vi "OdorSystem-V2.vi"() -> ()   [LabVIEW 2019]
doc: "Synchronize Correlated Digital Output with Analog Input Using NI-DAQmx \n\nOverview:\nThis example uses DAQmx to synchronize finite generation and acquisition of Correlated Digital Output with an Analog Input Task respectively.\n\nDescriptions:\nCorrelated I/O enables synchronization of on board digital I/O lines to a clock reference. Digital and Analog samples can be synchronized in time by sharing the AI clock as the source of your digital I/O clock. You may also use the Counter Output pulse as the Source of Digital Timing. Hence, set the Source for Digital Timing as ai/SampleClock.This example will work on any device that uses DAQmx and supports Correlated Digital I/O. To perform Correlated Digital I/O on 9172 Chassis, you need a Correlated Module in slot 1-4 of the chassis. \n\nRequirements:\n1. LabVIEW 2012 or compatible.\n2. NI-DAQmx 15.5.1 or compatible.\n\nInstructions:\n1. Set all the control values on the front panel corresponding to the physical channel to be used on the DAQ device.\n2. Run this VI.\n3. Monitor the analog input voltage measured and ramp signal generated from specified channels. \n\nBlock Diagram Steps:\n1. Creates channels to measure voltage and to generate digital signals \n2. Sets the source of the Sample Clock, the rate of the Sample Clock, and the number of samples to acquire or generate.\n3. Generates an array containing a ramp pattern and write to digital output lines.\n4. Transitions the tasks to running state to begin measuring and generating data.\n5. Reads the waveform from the analog input channel and waits for the digital output generation to complete.\n6. Clears the tasks.\n7. Displays any error occurs."
uses:
  StatesEnum.ctl
  <vilib>/DAQmx/write.llb/DAQmx Write (Digital 1D Bool NChan 1Samp 1Line).vi
  <vilib>/DAQmx/write.llb/DAQmx Write (Digital Wfm 1Chan NSamp).vi
  <vilib>/DAQmx/read.llb/DAQmx Read (Counter 1D U32 1Chan NSamp).vi
  <vilib>/DAQmx/read.llb/DAQmx Read (Digital 1D Bool 1Chan 1Samp).vi
  <vilib>/DAQmx/miscellaneous.llb/DAQmx Fill In Error Info.vi
  <vilib>/DAQmx/create/channels.llb/DAQmx Create Channel (CO-Pulse Generation-Frequency).vi
  <vilib>/DAQmx/configure/timing.llb/DAQmx Timing (Implicit).vi
  <vilib>/Waveform/DWDTOps.llb/Digital Pattern Generator (Single Value).vi
  <vilib>/Waveform/DWDTOps.llb/DWDT Append Digital Samples.vi
  <vilib>/DAQmx/create/channels.llb/DAQmx Create Channel (CI-Count Edges).vi
  <vilib>/DAQmx/configure/timing.llb/DAQmx Timing (Sample Clock).vi
  <vilib>/Waveform/DWDTOps.llb/DWDT Append Digital Signals.vi
  <vilib>/Waveform/DWDTOps.llb/DWDT Digital to Boolean Array.vi
  <vilib>/DAQmx/create/channels.llb/DAQmx Create Channel (DO-Digital Output).vi
  <vilib>/Waveform/DWDTOps.llb/DWDT Uncompress Digital.vi
  <resource>/objmgr/daqmx.rc
panel:
  in  "Use Default vavle":bool=TRUE
  in  "Selected default valve":u8(knob)=8 min=1 max=8 step=1 scale=1.0..8.0
  out "Framecount":u32
  in  "Image count filepath":path
  out "Experiment running":bool
  out "State":T1
  in  "Select experiment":enum32{"Single trial", "Trial series"}(tab)
  out "Time elapsed":dbl format="%.1f"
  in  "Start single trial":bool
  out "single trial done":bool
  in  "Select valve":u8(knob)=1 min=1 max=8 step=1 scale=1.0..8.0
  out "Pause elapsed time":dbl format="%#.1f"
  out "In between trials":bool
  out "Trial elapsed time":dbl format="%.1f"
  out "Total elapsed time":dbl format="%.1f"
  out "Estimated total time":dbl
  out "Current list index":i32
  out "Current Valve":u8
  in  "Time between trials":u16=10 min=1 max=900 step=1
  in  "Start trial series":bool
  in  "Valve order list":i8[](array[numeric]) min=1 max=8 step=1
  out "Digitaler output":digitalwaveform(graph)
  out "Stop Boolesch":bool
  in  "Total trial time":dbl=20.0 min=1.0 step=0.1
  in  "Valve opening Time":dbl=10.0 min=0.0 step=0.1
  in  "Valve delay":dbl=2.0 min=0.0 step=0.1
  in  "Stopp":bool
  out "Digital Waveform Graph":digitalwaveform(graph)
  # "All times are in second!"
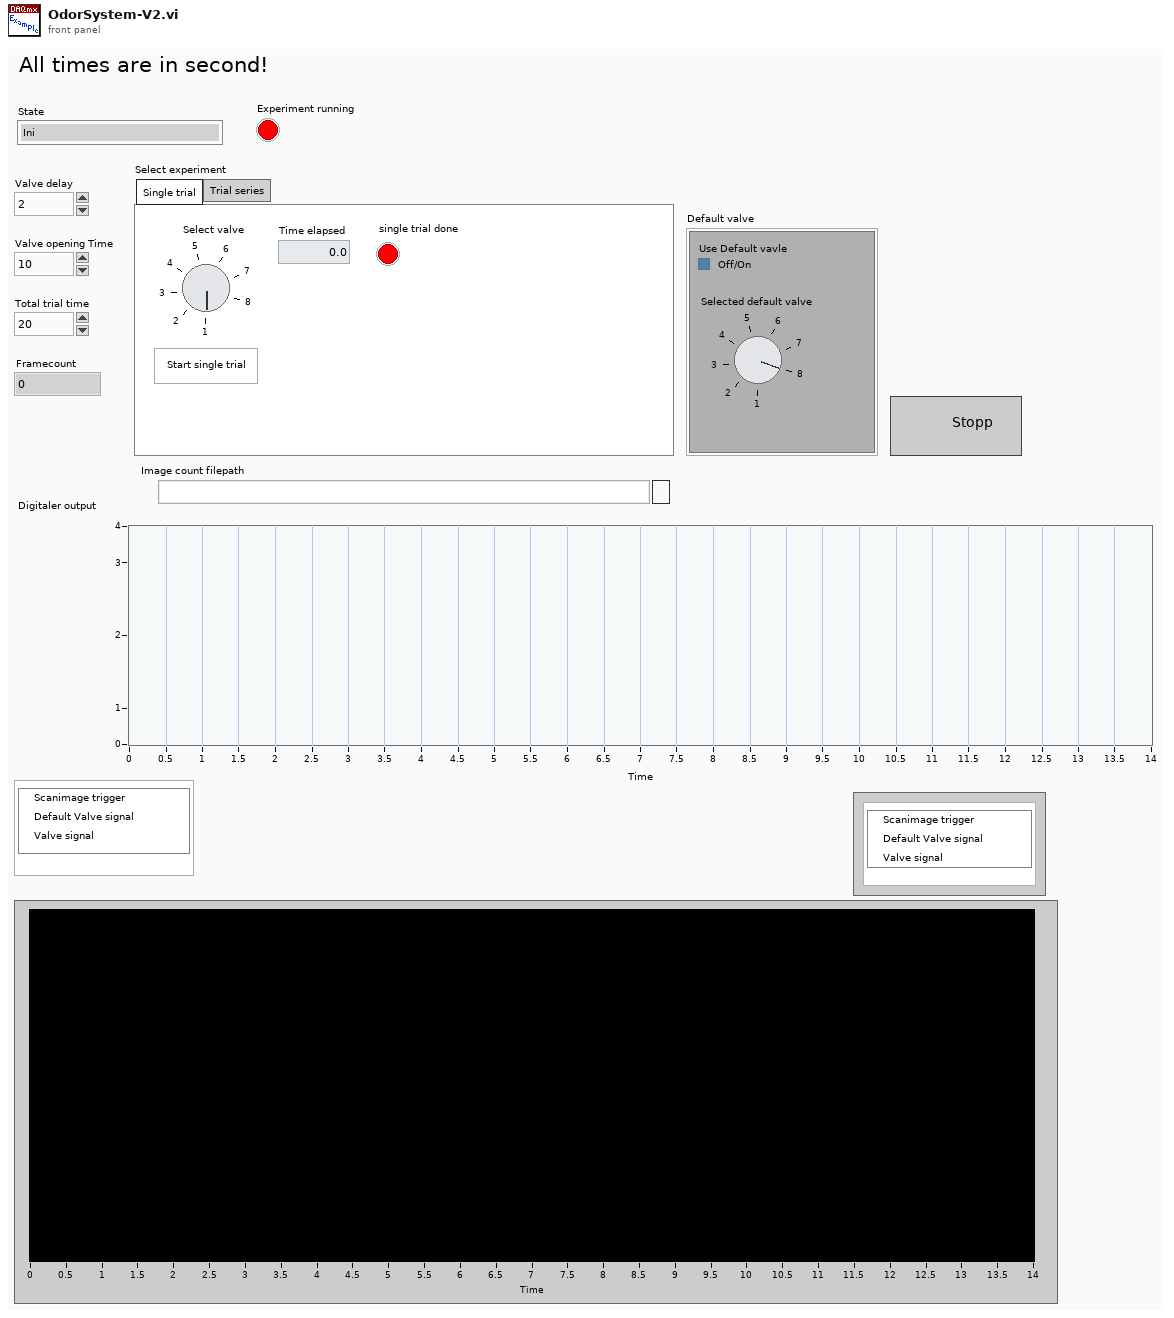
[diagram p1: front panel]
types:
  T1 = typedef "StatesEnum.ctl" = enum16{"Ini", "Standby", "Start Trial", "Start trial series", "Stop"}
  T2 = enum8{"Enabled", "Disabled", "Disabled and Grayed Out"}
  T3 = enum32{"Page Enabled", "Page Disabled", "Page Disabled & Grayed"}
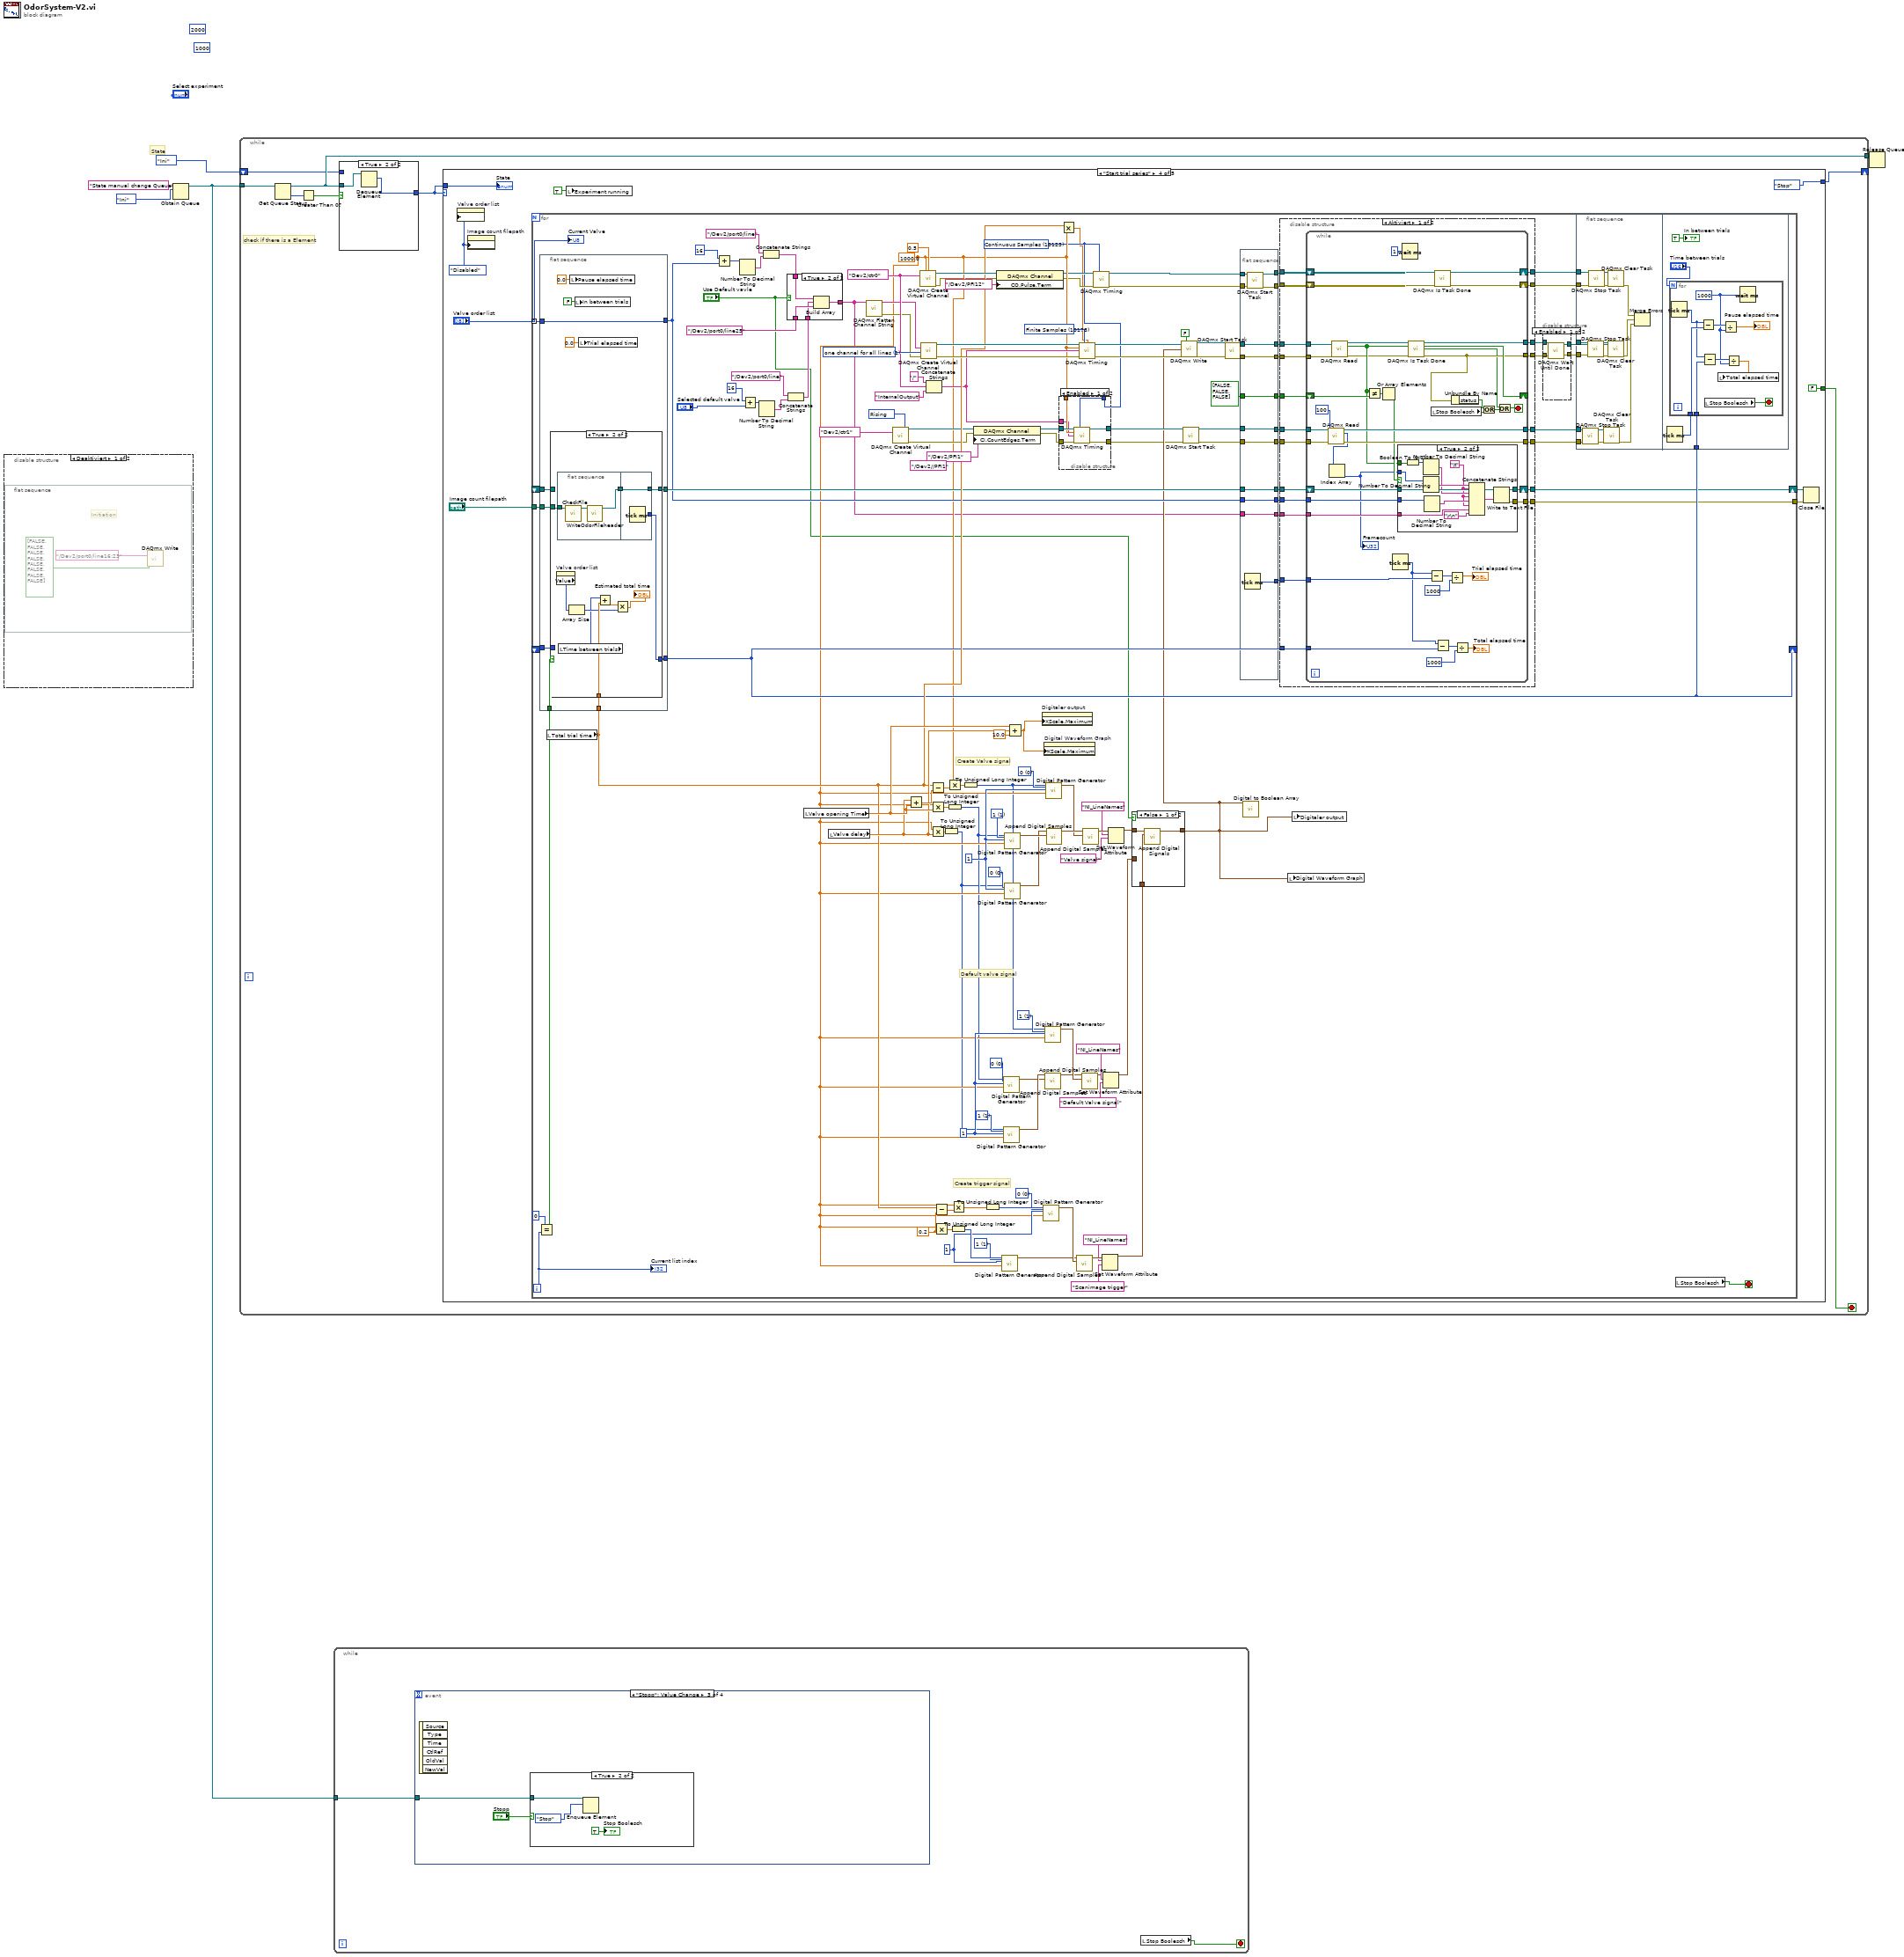
[diagram p0: block diagram]
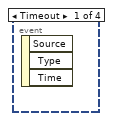
[diagram p3: hidden frame]
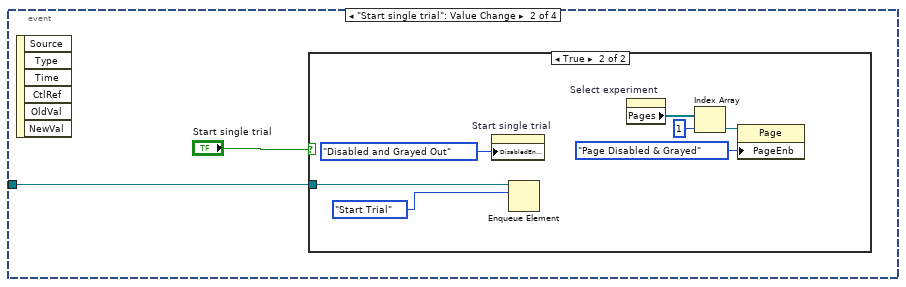
[diagram p4: hidden frame]
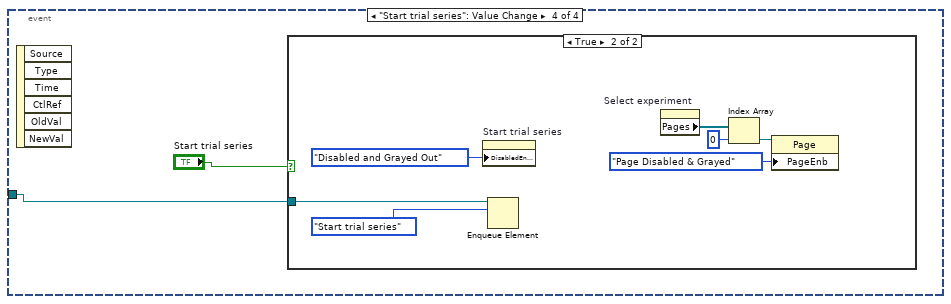
[diagram p7: hidden frame]
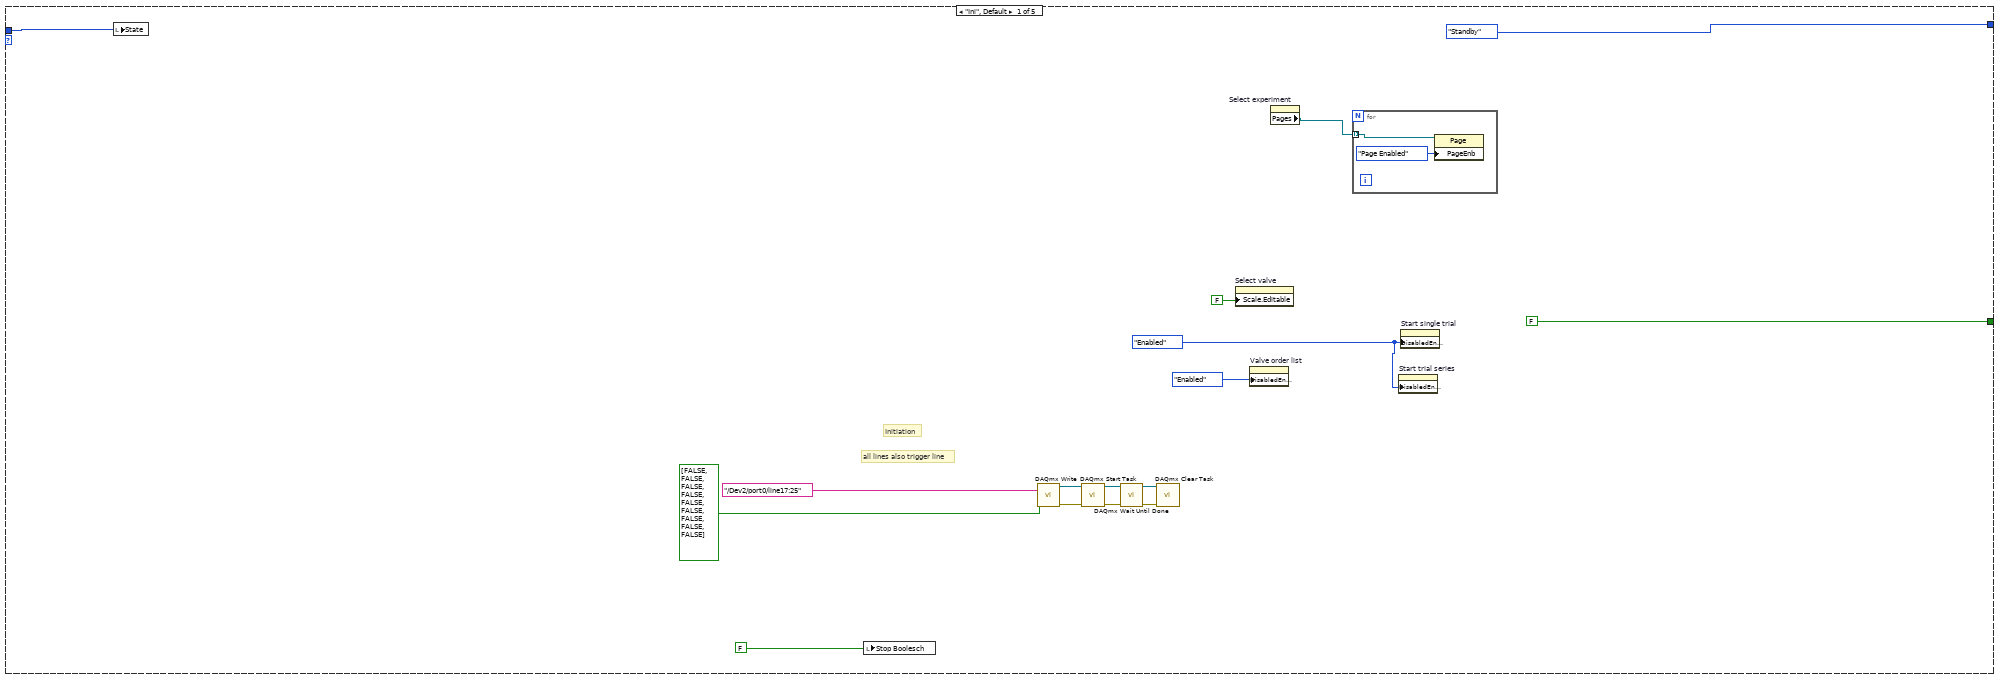
[diagram p10: hidden frame]
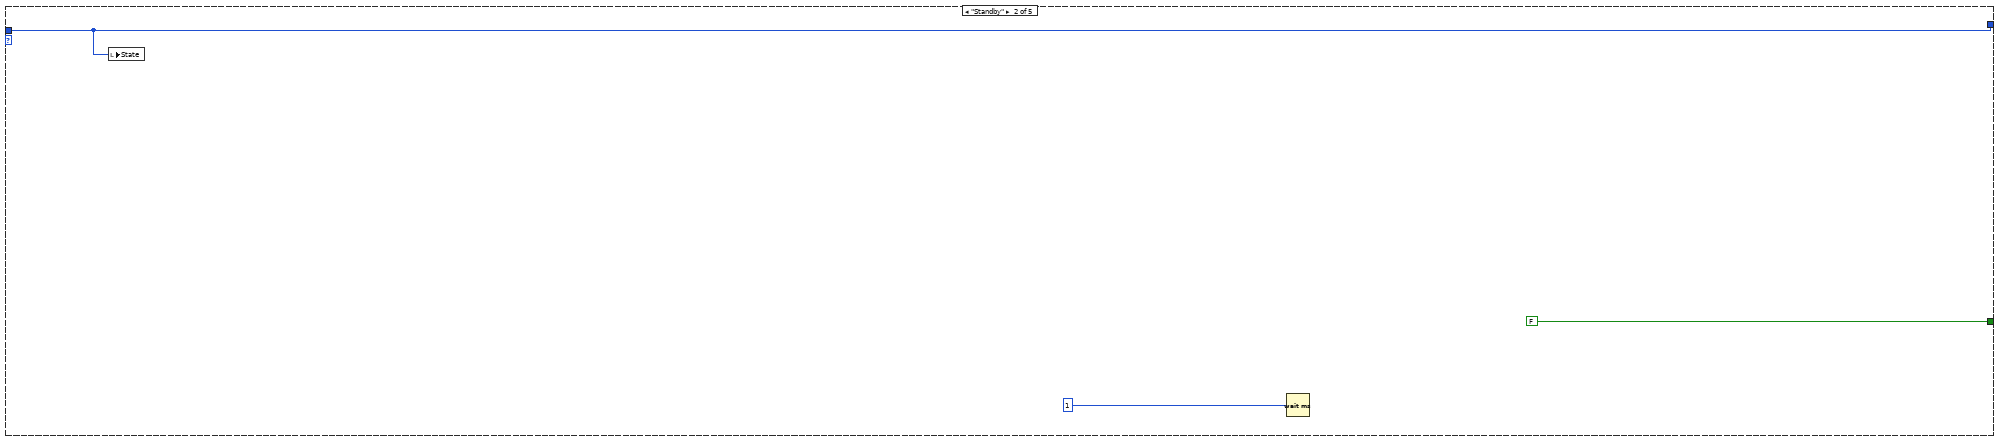
[diagram p11: hidden frame]
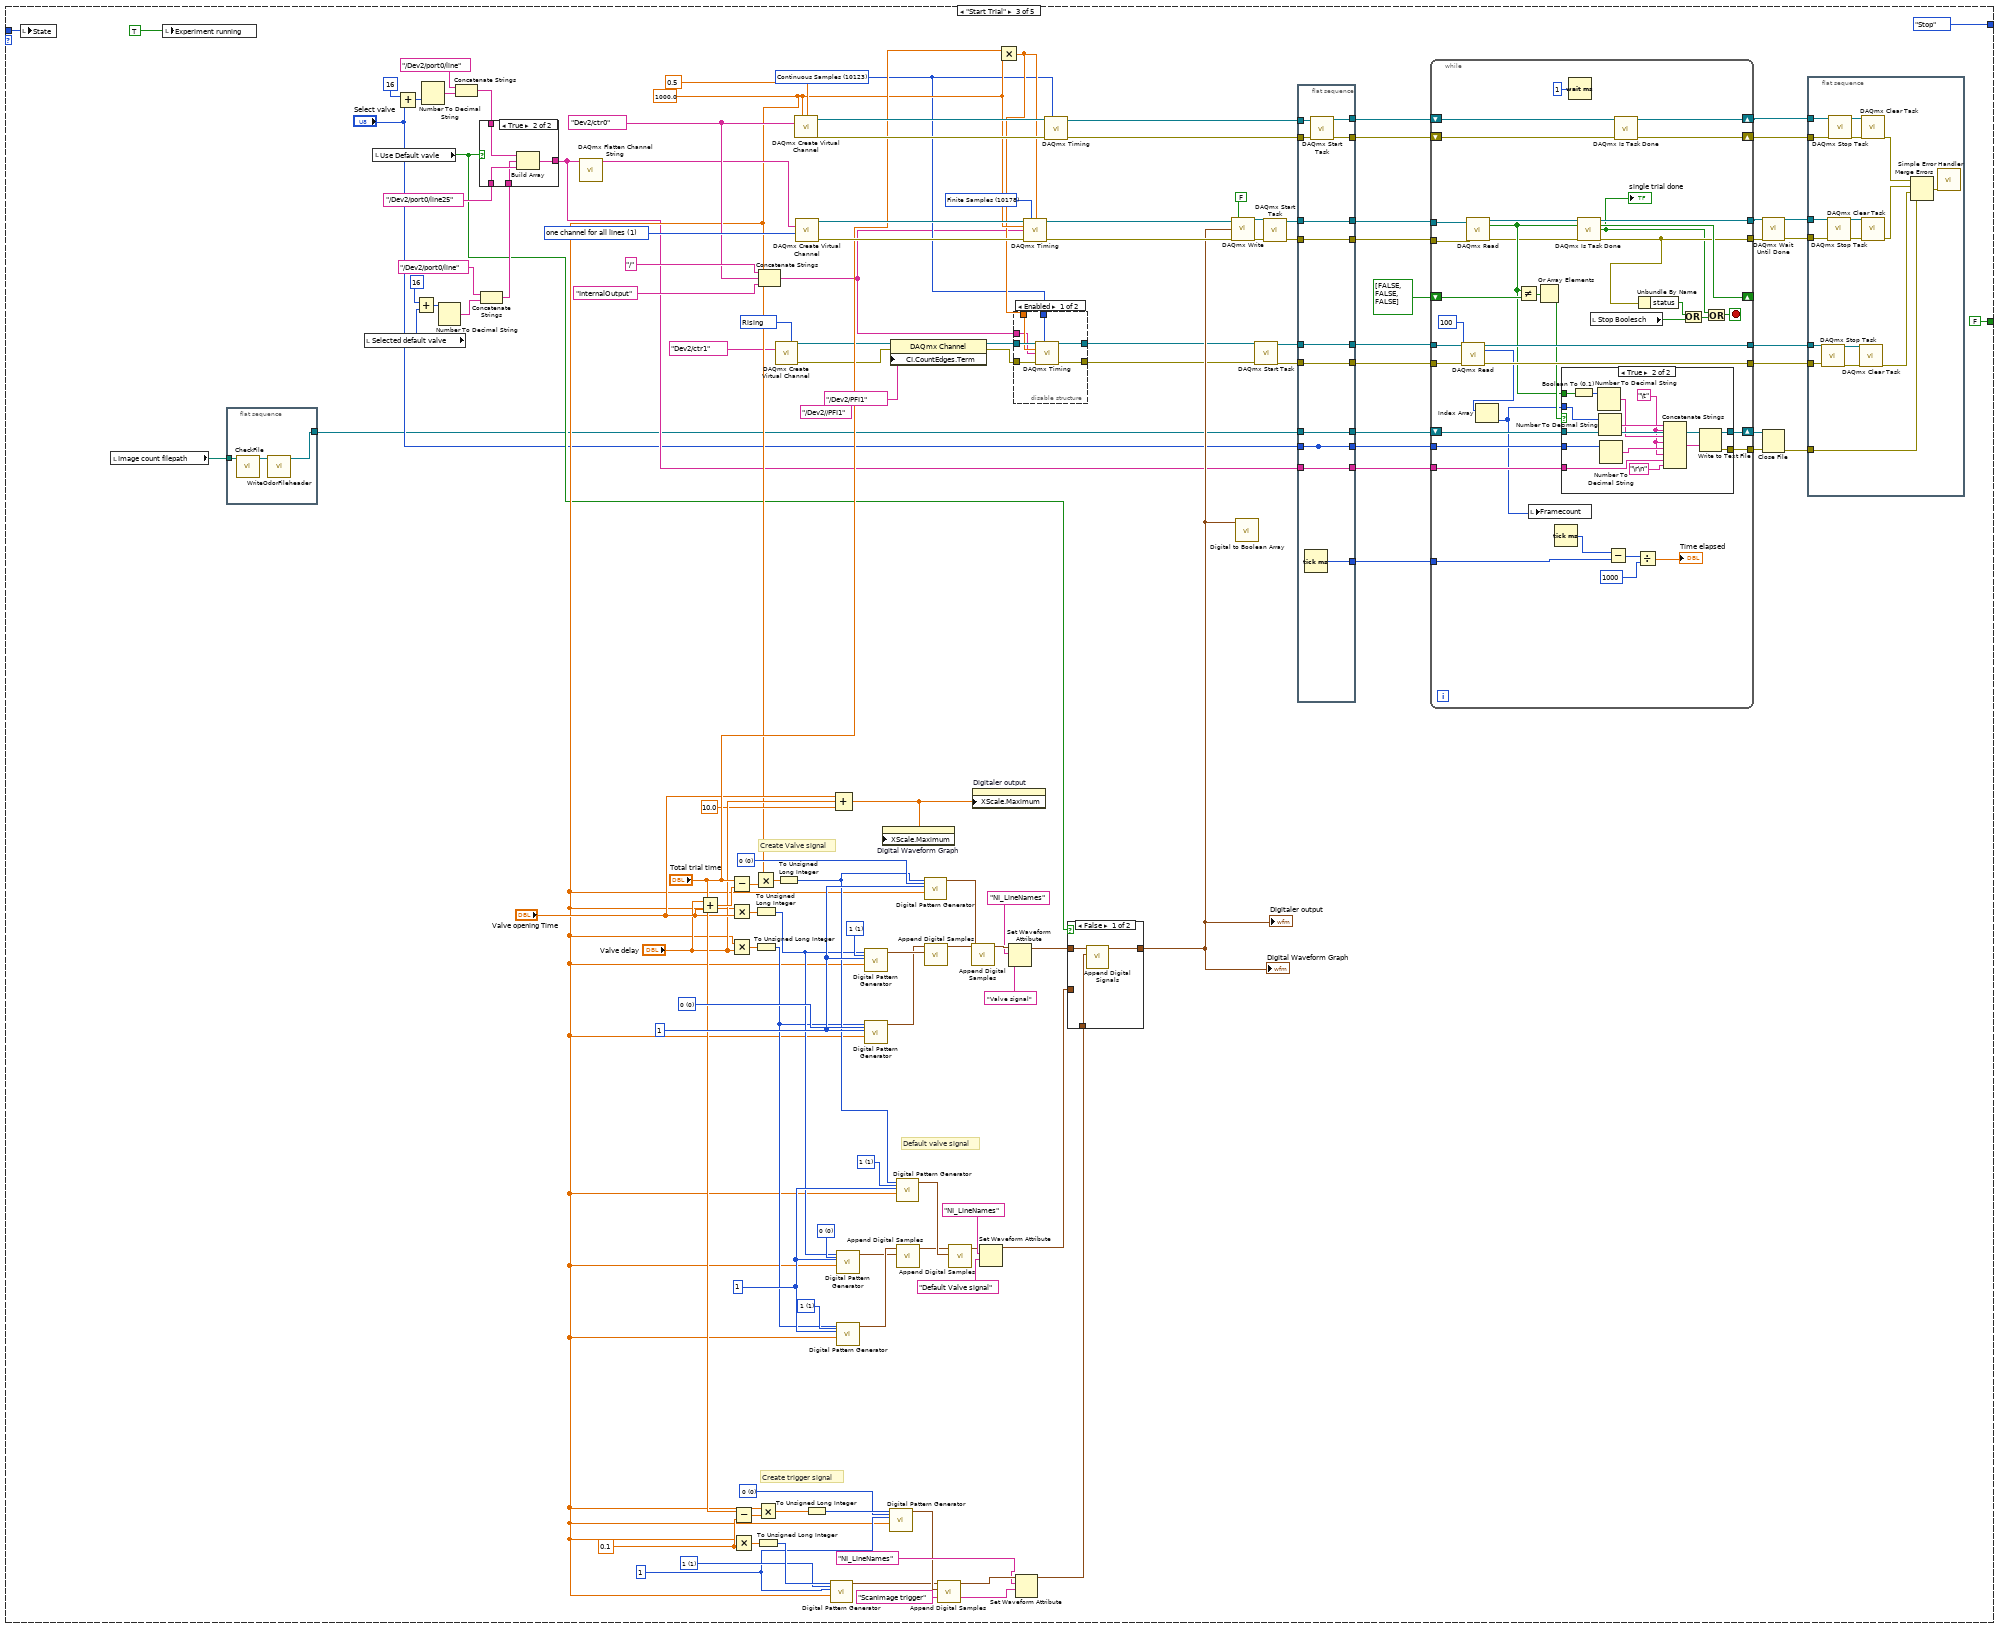
[diagram p12: hidden frame]
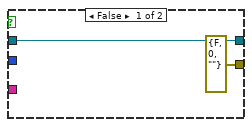
[diagram p13: hidden frame]
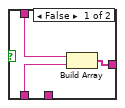
[diagram p14: hidden frame]
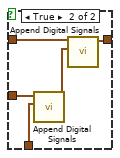
[diagram p16: hidden frame]
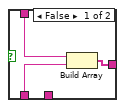
[diagram p17: hidden frame]
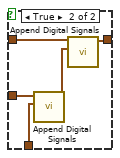
[diagram p18: hidden frame]
diagram:
  (unwired) u32 2000 ("number of samples")
  (unwired) u32 1000 ("number of samples")
  # "State"
  n1 = disable-structure shown="Deaktiviert" {
    frame Disabled {
      n2 = flat-sequence {
        frame #0 {
          # "Initiation"
          n3 = call-poly <vilib>:"DAQmx Write.vi"("task/channels in"="/Dev2/port0/line16:23" ("string"), "data"=bool[] [FALSE, FALSE, FALSE, FALSE, FALSE, FALSE, FALSE, FALSE]) -> ()  [unwired: 11 in, 3 out]
        }
      }
    }
    frame Enabled {
    }
  }
  n4 = Obtain Queue(name (unnamed)="State manual change Queue", element data type=StatesEnum."Ini" ("Enum")) -> (queue out=w4:refnum<queue>)  [unwired: 3 in, 2 out]
  n5 = while {
    tunnel: w4 -> [w13]
    tunnel: [w12] -> w3
    shift-right: [w8] -> _
    shift-left: StatesEnum."Ini" -> [w9]
    stop <- w11 stop-if-true
    # "check if there is a Element"
    n6 = Get Queue Status(queue=w13) -> (queue out=w12:refnum<queue>, # elements in queue=w15:i32)  [unwired: 2 in, 6 out]
    n7 = Greater Than 0?(x=w15) -> (x > 0?=w14:bool)
    n8 = case shown="True" w14 {
      tunnel: w12 -> [_ w18]
      tunnel: w9 -> [w16 _]
      tunnel: [w16 w17] -> w10
      frame False {
      }
      frame True {
        n9 = Dequeue Element(queue=w18) -> (element=w17:T1)  [unwired: 2 in, 3 out]
      }
    }
    n10 = case shown="\"Start trial series\"" w10 {
      tunnel: w10 -> [w29 w37 w109 w286 w604]
      tunnel: [FALSE ("Stop Boolesch") FALSE ("Stop Boolesch") FALSE ("Stop Boolesch") FALSE ("Stop Boolesch") w606] -> w11
      tunnel: [StatesEnum."Standby" ("Enum") w37 StatesEnum."Stop" ("Enum") StatesEnum."Stop" ("Enum") StatesEnum."Standby" ("Enum")] -> w8
      frame "Ini", Default {
        w22 = T2."Enabled" ("Deaktiviert")
        # "all lines also trigger line"
        # "Initiation"
        n11 = local write "State"(w29) -> ()
        n12 = local write "Stop Boolesch"(FALSE ("Stop Boolesch")) -> ()
        n13 = call-poly <vilib>:"DAQmx Write.vi"("task/channels in"="/Dev2/port0/line17:25" ("string"), "data"=bool[] [FALSE, FALSE, FALSE, FALSE, FALSE, FALSE, FALSE, FALSE, FALSE]) -> ("task out"=w24:refnum<k21>, "error out"=w23:errorcluster)  [unwired: 11 in, 1 out]
        n14 = call <vilib>:"DAQmx Start Task.vi"("task/channels in"=w24, "error in"=w23) -> ("task out"=w28:refnum<k21>, "error out"=w26:errorcluster)  [unwired: 12 in]
        n15 = call <vilib>:"DAQmx Wait Until Done.vi"("task/channels in"=w28, "error in"=w26) -> ("task out"=w27:refnum<k21>, "error out"=w25:errorcluster)  [unwired: 12 in]
        n16 = call <vilib>:"DAQmx Clear Task.vi"("task in"=w27, "error in"=w25) -> ()  [unwired: 13 in, 1 out]
        n17 = property on="Select valve" class="Knob (strict)"("Scale.Editable"=FALSE ("Skala.Editierbar")) -> ()  [unwired: 2 in, 2 out]
        n18 = property on="Valve order list" class="Arr (strict)"("DisabledEnum"=T2."Enabled" ("Deaktiviert")) -> ()  [unwired: 2 in, 2 out]
        n19 = property on="Select experiment" class="TabCtl (strict)"() -> ("Pages"=w20:refnum<vi>[])  [unwired: 2 in, 2 out]
        n20 = for {
          tunnel: w20 -> [w35] mode=indexing
          n21 = property class="Page"(reference=w35, "PageEnb"=T3."Page Enabled" ("Aktiv-Status der Seite")) -> ()  [unwired: 1 in, 2 out]
        }
        n22 = property on="Start trial series" class="Bool"("DisabledEnum"=w22) -> ()  [unwired: 2 in, 2 out]
        n23 = property on="Start single trial" class="Bool"("DisabledEnum"=w22) -> ()  [unwired: 2 in, 2 out]
      }
      frame "Standby" {
        n24 = local write "State"(w37) -> ()
        n25 = Wait (ms)(milliseconds to wait=u32 1 ("Zu wartende ms")) -> ()  [unwired: 1 out]
      }
      frame "Start Trial" {
        w77 = 10178 items=["Finite Samples"=10178, "Continuous Samples"=10123, "Hardware Timed Single Point"=12522] ("sample mode")
        (unwired) "/Dev2//PFI1" ("string")
        w87 = 10280 items=["Rising"=10280, "Falling"=10171] ("edge")
        w97 = u32 1 ("number of signals")
        w100 = u8 1 items=["0", "1", "Z", "L", "H", "X", "T", "V"] ("value")
        w99 = u8 0 items=["0", "1", "Z", "L", "H", "X", "T", "V"] ("value")
        w98 = u8 1 items=["0", "1", "Z", "L", "H", "X", "T", "V"] ("value")
        w129 = 0.1 ("y")
        w132 = u32 1 ("number of signals")
        w134 = u8 0 items=["0", "1", "Z", "L", "H", "X", "T", "V"] ("value")
        w133 = u8 1 items=["0", "1", "Z", "L", "H", "X", "T", "V"] ("value")
        w149 = tag "Dev2/ctr0" ("counter")
        w93 = 1000.0 ("frequency")
        w153 = u32 1 ("number of signals")
        w154 = u8 0 items=["0", "1", "Z", "L", "H", "X", "T", "V"] ("value")
        w155 = u8 1 items=["0", "1", "Z", "L", "H", "X", "T", "V"] ("value")
        w156 = u8 0 items=["0", "1", "Z", "L", "H", "X", "T", "V"] ("value")
        w164 = 1 items=["one channel for each line", "one channel for all lines"] ("line grouping")
        w78 = 10123 items=["Finite Samples"=10178, "Continuous Samples"=10123] ("sample mode")
        # "Default valve signal"
        # "Create trigger signal"
        # "Create Valve signal"
        n26 = local write "State"(w109) -> ()
        n27 = local read "Image count filepath"() -> (w48:path)
        n28 = local write "Experiment running"(TRUE ("Experiment running")) -> ()
        n29 = flat-sequence {
          tunnel: w48 -> [w190]
          tunnel: [w188] -> w49
          frame #0 {
            n30 = call "CheckFile.vi"("Image count filepath"=w190) -> ("Byte Stream File out"=w189:refnum<file>)  [unwired: 10 in]
            n31 = call "WriteOdorFileheader.vi"("Byte Stream File in"=w189) -> ("Byte Stream File out"=w188:refnum<file>)  [unwired: 10 in]
          }
        }
        n32 = local read "Selected default valve"() -> (w67:u8)
        n33 = local read "Use Default vavle"() -> (w68:bool)
        n34 = Add(x=i8 16, y="Select valve") -> (x+y=w141:u8)
        n35 = Add(x=i8 16, y=w67) -> (x+y=w74:u8)
        n36 = Number To Decimal String(number=w141) -> (decimal integer string=w142:string)  [unwired: 1 in]
        n37 = Number To Decimal String(number=w74) -> (decimal integer string=w73:string)  [unwired: 1 in]
        n38 = Concatenate Strings("/Dev2/port0/line" ("string"), w142) -> (w71:string)
        n39 = Concatenate Strings("/Dev2/port0/line" ("string"), w73) -> (w69:string)
        n40 = case shown="True" w68 {
          tunnel: w71 -> [w246 w249]
          tunnel: "/Dev2/port0/line25" ("string") -> [w245 w248]
          tunnel: [w244 w250] -> w52
          tunnel: w69 -> [_ w247]
          frame False {
            n41 = Build Array(w246, w245) -> (w244:string[])
          }
          frame True {
            n42 = Build Array(w249, w247, w248) -> (w250:string[])
          }
        }
        n43 = call <vilib>:"DAQmx Flatten Channel String.vi"("names in"=w52) -> ("names out"=w131:string)  [unwired: 13 in, 1 out]
        n44 = Add(x="Valve delay", y="Valve opening Time") -> (x+y=w145:dbl)
        n45 = Subtract(x="Total trial time", y=w145) -> (x-y=w144:dbl)
        n46 = Multiply(x=w93, y="Valve opening Time") -> (x*y=w147:dbl)
        n47 = Multiply(x=w93, y="Valve delay") -> (x*y=w148:dbl)
        n48 = Subtract(x="Total trial time", y=w129) -> (x-y=w139:dbl)
        n49 = Multiply(x=w93, y=w129) -> (x*y=w135:dbl)
        n50 = Multiply(x=w93, y=w144) -> (x*y=w146:dbl)
        n51 = To Unsigned Long Integer(number=w147) -> (unsigned 32bit integer=w95:u32)
        n52 = To Unsigned Long Integer(number=w148) -> (unsigned 32bit integer=w94:u32)
        n53 = Multiply(x=w93, y=w139) -> (x*y=w137:dbl)
        n54 = To Unsigned Long Integer(number=w135) -> (unsigned 32bit integer=w136:u32)
        n55 = Concatenate Strings("/", w149, "InternalOutput" ("string")) -> (w76:string)
        n56 = call-poly <vilib>:"DAQmx Create Virtual Channel.vi"("edge"=w87, "counter"=tag "Dev2/ctr1") -> ("task out"=w85:refnum<k21>, "error out"=w82:errorcluster)  [unwired: 12 in]
        n57 = To Unsigned Long Integer(number=w146) -> (unsigned 32bit integer=w96:u32)
        n58 = call-poly <vilib>:"DAQmx Create Virtual Channel.vi"("frequency"=w93, "duty cycle"=0.5, "counter"=w149) -> ("task out"=w167:refnum<k21>, "error out"=w168:errorcluster)  [unwired: 11 in]
        n59 = call-poly <vilib>:"DAQmx Create Virtual Channel.vi"("lines"=w131, "line grouping"=w164) -> ("task out"=w170:refnum<k21>, "error out"=w169:errorcluster)  [unwired: 12 in]
        n60 = To Unsigned Long Integer(number=w137) -> (unsigned 32bit integer=w138:u32)
        n61 = call-poly <vilib>:"Digital Pattern Generator.vi"("value"=w133, "sample rate"=w93, "number of signals"=w132, "number of samples"=w136) -> ("digital waveform"=w117:digitalwaveform)  [unwired: 6 in, 1 out]
        n62 = Compound Arithmetic op=ADD("Valve opening Time", "Valve delay", 10.0 ("Wert")) -> (w110:dbl)
        n63 = call-poly <vilib>:"Digital Pattern Generator.vi"("value"=w99, "sample rate"=w93, "number of signals"=w97, "number of samples"=w95) -> ("digital waveform"=w104:digitalwaveform)  [unwired: 6 in, 1 out]
        n64 = call-poly <vilib>:"Digital Pattern Generator.vi"("value"=w98, "sample rate"=w93, "number of signals"=w97, "number of samples"=w94) -> ("digital waveform"=w105:digitalwaveform)  [unwired: 6 in, 1 out]
        n65 = call-poly <vilib>:"Digital Pattern Generator.vi"("value"=w155, "sample rate"=w93, "number of signals"=w153, "number of samples"=w95) -> ("digital waveform"=w122:digitalwaveform)  [unwired: 6 in, 1 out]
        n66 = call-poly <vilib>:"Digital Pattern Generator.vi"("value"=w156, "sample rate"=w93, "number of signals"=w153, "number of samples"=w94) -> ("digital waveform"=w121:digitalwaveform)  [unwired: 6 in, 1 out]
        n67 = property on="Digital Waveform Graph" class="DigitalGraph (strict)"("XScale.Maximum"=w110) -> ()  [unwired: 2 in, 2 out]
        n68 = call-poly <vilib>:"Digital Pattern Generator.vi"("value"=w134, "sample rate"=w93, "number of signals"=w132, "number of samples"=w138) -> ("digital waveform"=w118:digitalwaveform)  [unwired: 6 in, 1 out]
        n69 = property class="DAQmx Channel"(reference=w85, error in=w82, "CI.CountEdges.Term"=tag "/Dev2/PFI1") -> (reference out=w84:refnum<k21>, error out=w83:errorcluster)
        n70 = call-poly <vilib>:"Digital Pattern Generator.vi"("value"=w100, "sample rate"=w93, "number of signals"=w97, "number of samples"=w96) -> ("digital waveform"=w107:digitalwaveform)  [unwired: 6 in, 1 out]
        n71 = call-poly <vilib>:"Append Digital Samples.vi"("digital waveform B"=w104, "digital waveform A"=w105) -> ("digital waveform out"=w106:digitalwaveform)  [unwired: 8 in, 1 out]
        n72 = call-poly <vilib>:"Digital Pattern Generator.vi"("value"=w154, "sample rate"=w93, "number of signals"=w153, "number of samples"=w96) -> ("digital waveform"=w119:digitalwaveform)  [unwired: 6 in, 1 out]
        n73 = call-poly <vilib>:"Append Digital Samples.vi"("digital waveform B"=w122, "digital waveform A"=w121) -> ("digital waveform out"=w120:digitalwaveform)  [unwired: 8 in, 1 out]
        n74 = call-poly <vilib>:"Append Digital Samples.vi"("digital waveform B"=w118, "digital waveform A"=w117) -> ("digital waveform out"=w128:digitalwaveform)  [unwired: 8 in, 1 out]
        n75 = call-poly <vilib>:"Append Digital Samples.vi"("digital waveform B"=w107, "digital waveform A"=w106) -> ("digital waveform out"=w101:digitalwaveform)  [unwired: 8 in, 1 out]
        n76 = call-poly <vilib>:"Append Digital Samples.vi"("digital waveform B"=w119, "digital waveform A"=w120) -> ("digital waveform out"=w125:digitalwaveform)  [unwired: 8 in, 1 out]
        n77 = property on="Digitaler output" class="DigitalGraph (strict)"("XScale.Maximum"=w110) -> ()  [unwired: 2 in, 2 out]
        n78 = Set Waveform Attribute(5:"Default Valve signal", 6:"NI_LineNames" ("name"), 7:w101) -> (3:w89:digitalwaveform)  [unwired: 1 in, 2 out]
        n79 = Multiply(x="Total trial time", y=w93) -> (x*y=w79:dbl)
        n80 = Set Waveform Attribute(5:"Valve signal", 6:"NI_LineNames" ("name"), 7:w125) -> (3:w92:digitalwaveform)  [unwired: 1 in, 2 out]
        n81 = disable-structure shown="Enabled" {
          disable-tunnel: w84 -> [w257 w259]
          disable-tunnel: w79 -> [w256 _]
          disable-tunnel: w76 -> [w255 _]
          disable-tunnel: w83 -> [w254 w258]
          disable-tunnel: [w253 w259] -> w86
          disable-tunnel: [w252 w258] -> w80
          disable-tunnel: w78 -> [w251 _]
          frame Enabled {
            n82 = call-poly <vilib>:"DAQmx Timing.vi"("task/channels in"=w257, "sample mode"=w251, "rate"=w256, "source"=w255, "error in"=w254) -> ("task out"=w253:refnum<k21>, "error out"=w252:errorcluster)  [unwired: 9 in]
          }
          frame Disabled {
          }
        }
        n83 = Set Waveform Attribute(5:"Scanimage trigger", 6:"NI_LineNames" ("name"), 7:w128) -> (3:w90:digitalwaveform)  [unwired: 1 in, 2 out]
        n84 = call-poly <vilib>:"DAQmx Timing.vi"("task/channels in"=w170, "sample mode"=w77, "samples per channel"=w79, "rate"=w93, "source"=w76, "error in"=w169) -> ("task out"=w161:refnum<k21>, "error out"=w160:errorcluster)  [unwired: 8 in]
        n85 = call-poly <vilib>:"DAQmx Timing.vi"("task/channels in"=w167, "sample mode"=w78, "error in"=w168) -> ("task out"=w165:refnum<k21>, "error out"=w166:errorcluster)  [unwired: 11 in]
        n86 = case shown="False" w68 {
          tunnel: w92 -> [w262 w267]
          tunnel: w90 -> [w261 w265]
          tunnel: [w260 w266] -> w91
          tunnel: w89 -> [_ w264]
          frame False {
            n87 = call-poly <vilib>:"Append Digital Signals.vi"("digital waveform (low bits)"=w261, "digital waveform (high bits)"=w262) -> ("digital waveform out"=w260:digitalwaveform)  [unwired: 8 in, 1 out]
          }
          frame True {
            n88 = call-poly <vilib>:"Append Digital Signals.vi"("digital waveform (low bits)"=w265, "digital waveform (high bits)"=w264) -> ("digital waveform out"=w263:digitalwaveform)  [unwired: 8 in, 1 out]
            n89 = call-poly <vilib>:"Append Digital Signals.vi"("digital waveform (low bits)"=w263, "digital waveform (high bits)"=w267) -> ("digital waveform out"=w266:digitalwaveform)  [unwired: 8 in, 1 out]
          }
        }
        "Digital Waveform Graph" <- w91
        "Digitaler output" <- w91
        n90 = call-poly <vilib>:"DAQmx Write.vi"("task/channels in"=w161, "auto start"=FALSE, "data"=w91, "error in"=w160) -> ("task out"=w159:refnum<k21>, "error out"=w158:errorcluster)  [unwired: 9 in, 1 out]
        n91 = call-poly <vilib>:"Digital to Boolean Array.vi"("digital waveform"=w91) -> ()  [unwired: 9 in, 2 out]
        n92 = call <vilib>:"DAQmx Start Task.vi"("task/channels in"=w86, "error in"=w80) -> ("task out"=w60:refnum<k21>, "error out"=w59:errorcluster)  [unwired: 12 in]
        n93 = call <vilib>:"DAQmx Start Task.vi"("task/channels in"=w159, "error in"=w158) -> ("task out"=w163:refnum<k21>, "error out"=w162:errorcluster)  [unwired: 12 in]
        n94 = flat-sequence {
          tunnel: [w279] -> w66
          tunnel: [w278] -> w65
          tunnel: w166 -> [w277]
          tunnel: w165 -> [w276]
          tunnel: [w275] -> w64
          tunnel: w163 -> [w275]
          tunnel: [w274] -> w63
          tunnel: w162 -> [w274]
          tunnel: [w273] -> w56
          tunnel: [w272] -> w58
          tunnel: w60 -> [w272]
          tunnel: [w271] -> w57
          tunnel: w59 -> [w271]
          tunnel: [w270] -> w55
          tunnel: w52 -> [w270]
          tunnel: [w268] -> w54
          tunnel: [w268] -> _
          tunnel: [w269] -> w53
          tunnel: w49 -> [w269]
          tunnel: "Select valve" -> [w268]
          frame #0 {
            n95 = Tick Count (ms)() -> (millisecond timer value=w273:u32)
            n96 = call <vilib>:"DAQmx Start Task.vi"("task/channels in"=w276, "error in"=w277) -> ("task out"=w279:refnum<k21>, "error out"=w278:errorcluster)  [unwired: 12 in]
          }
        }
        n97 = while {
          shift-right: [w224] -> w62
          shift-left: w66 -> [w226]
          shift-right: [w223] -> w42
          shift-left: w65 -> [w225]
          tunnel: w64 -> [w222]
          tunnel: w63 -> [w213]
          tunnel: [w199] -> w61
          tunnel: [w197] -> w40
          tunnel: w56 -> [w218]
          tunnel: w58 -> [w212]
          tunnel: w57 -> [w210]
          tunnel: [w211] -> w45
          tunnel: [w209] -> w44
          shift-right: [w205] -> _
          shift-left: bool[] [FALSE, FALSE, FALSE] ("data") -> [w208]
          shift-right: [w203] -> w47
          shift-left: w53 -> [w204]
          tunnel: w55 -> [w202]
          tunnel: w54 -> [w201]
          tunnel: [w200] -> w46
          stop <- w219 stop-if-true
          n98 = call-poly <vilib>:"DAQmx Read.vi"("task/channels in"=w212, "number of samples per channel"=100, "error in"=w210) -> ("task out"=w211:refnum<k21>, "data"=w192:u32[], "error out"=w209:errorcluster)  [unwired: 10 in]
          n99 = call-poly <vilib>:"DAQmx Read.vi"("task/channels in"=w222, "error in"=w213) -> ("task out"=w214:refnum<k21>, "data"=w205:bool[], "error out"=w198:errorcluster)  [unwired: 11 in]
          n100 = Index Array(array=w192) -> (element=w193:u32)  [unwired: 1 in]
          n101 = Not Equal?(x=w205, y=w208) -> (x != y?=w207:bool[])
          n102 = local write "Framecount"(w193) -> ()
          n103 = Or Array Elements(Boolean array=w207) -> (logical OR=w206:bool)
          n104 = Tick Count (ms)() -> (millisecond timer value=w217:u32)
          n105 = case shown="True" w206 {
            tunnel: w205 -> [_ w240]
            tunnel: w193 -> [_ w238]
            tunnel: w204 -> [w229 w242]
            tunnel: [w229 w241] -> w203
            tunnel: w202 -> [_ w232]
            tunnel: w201 -> [_ w235]
            tunnel: [errorcluster {"status"=FALSE, "code"=0, "source"=""} ("error out") w231] -> w200
            frame False {
            }
            frame True {
              w233 = "\t"
              n106 = Boolean To (0,1)(Boolean=w240) -> (0, 1=w239:i16[])
              n107 = Number To Decimal String(number=w239) -> (decimal integer string=w236:string[])  [unwired: 1 in]
              n108 = Number To Decimal String(number=w238) -> (decimal integer string=w237:string)  [unwired: 1 in]
              n109 = Number To Decimal String(number=w235) -> (decimal integer string=w234:string)  [unwired: 1 in]
              n110 = Concatenate Strings(w237, w233, w236, w233, w234, w233, w232, "\r\n") -> (w243:string)
              n111 = Write to Text File(file (use dialog)=w242, text=w243) -> (refnum out=w241:refnum<file>, error out=w231:errorcluster)  [unwired: 2 in, 1 out]
            }
          }
          n112 = Wait (ms)(milliseconds to wait=u32 1 ("Zu wartende ms")) -> ()  [unwired: 1 out]
          n113 = call <vilib>:"DAQmx Is Task Done.vi"("task/channels in"=w214, "error in"=w198) -> ("task out"=w199:refnum<k21>, "task done?"=w195:bool, "error out"=w197:errorcluster)  [unwired: 11 in]
          "single trial done" <- w195
          n114 = local read "Stop Boolesch"() -> (w196:bool)
          n115 = Subtract(x=w217, y=w218) -> (x-y=w216:u32)
          n116 = call <vilib>:"DAQmx Is Task Done.vi"("task/channels in"=w226, "error in"=w225) -> ("task out"=w224:refnum<k21>, "error out"=w223:errorcluster)  [unwired: 11 in, 1 out]
          n117 = Divide(x=w216, y=u32 1000 ("x")) -> (x/y=→"Time elapsed":dbl)
          n118 = Unbundle By Name(w197) -> ("status"=w220:bool)
          n119 = Or(x=w220, y=w196) -> (x .or. y?=w227:bool)
          n120 = Or(x=w195, y=w227) -> (x .or. y?=w219:bool)
        }
        n121 = call <vilib>:"DAQmx Wait Until Done.vi"("task/channels in"=w61, "error in"=w40) -> ("task out"=w113:refnum<k21>, "error out"=w43:errorcluster)  [unwired: 12 in]
        n122 = Close File(refnum=w47, error in=w46) -> (error out=w41:errorcluster)  [unwired: 1 out]
        n123 = flat-sequence {
          tunnel: w113 -> [w184]
          tunnel: w62 -> [w183]
          tunnel: w45 -> [w181]
          tunnel: w44 -> [w180]
          tunnel: w43 -> [w176]
          tunnel: w42 -> [w173]
          tunnel: w41 -> [w171]
          frame #0 {
            n124 = call <vilib>:"DAQmx Stop Task.vi"("task/channels in"=w181, "error in"=w180) -> ("task out"=w182:refnum<k21>, "error out"=w179:errorcluster)  [unwired: 12 in]
            n125 = call <vilib>:"DAQmx Stop Task.vi"("task/channels in"=w184, "error in"=w176) -> ("task out"=w177:refnum<k21>, "error out"=w175:errorcluster)  [unwired: 12 in]
            n126 = call <vilib>:"DAQmx Stop Task.vi"("task/channels in"=w183, "error in"=w173) -> ("task out"=w174:refnum<k21>, "error out"=w172:errorcluster)  [unwired: 12 in]
            n127 = call <vilib>:"DAQmx Clear Task.vi"("task in"=w182, "error in"=w179) -> ("error out"=w178:errorcluster)  [unwired: 13 in]
            n128 = call <vilib>:"DAQmx Clear Task.vi"("task in"=w174, "error in"=w172) -> ("error out"=w187:errorcluster)  [unwired: 13 in]
            n129 = call <vilib>:"DAQmx Clear Task.vi"("task in"=w177, "error in"=w175) -> ("error out"=w186:errorcluster)  [unwired: 13 in]
            n130 = Merge Errors(w187, w186, w178, w171) -> (w185:errorcluster)
            n131 = call <vilib>:"Simple Error Handler.vi"("error in (no error)"=w185) -> ()  [unwired: 4 in, 5 out]
          }
        }
      }
      frame "Start trial series" {
        w282 = T2."Disabled" ("Deaktiviert")
        n132 = property on="Valve order list" class="Arr (strict)"("DisabledEnum"=w282) -> ()  [unwired: 2 in, 2 out]
        n133 = property on="Image count filepath" class="Path"("DisabledEnum"=w282) -> ()  [unwired: 2 in, 2 out]
        n134 = for {
          tunnel: "Valve order list" -> [w357] mode=indexing
          shift-right: [w353] -> _
          shift-left: _ -> [w355]
          tunnel: "Image count filepath" -> [w337]
          shift-right: [w336] -> w281
          shift-left: _ -> [w335]
          tunnel: [w334] -> w280
          i -> [w362]
          stop <- w366 stop-if-true
          w290 = 10178 items=["Finite Samples"=10178, "Continuous Samples"=10123, "Hardware Timed Single Point"=12522] ("sample mode")
          w319 = u32 1 ("number of signals")
          w322 = u8 1 items=["0", "1", "Z", "L", "H", "X", "T", "V"] ("value")
          w321 = u8 0 items=["0", "1", "Z", "L", "H", "X", "T", "V"] ("value")
          w320 = u8 1 items=["0", "1", "Z", "L", "H", "X", "T", "V"] ("value")
          (unwired) "/Dev2//PFI1" ("string")
          w350 = 10280 items=["Rising"=10280, "Falling"=10171] ("edge")
          w383 = 0.2 ("y")
          w385 = u32 1 ("number of signals")
          w387 = u8 0 items=["0", "1", "Z", "L", "H", "X", "T", "V"] ("value")
          w386 = u8 1 items=["0", "1", "Z", "L", "H", "X", "T", "V"] ("value")
          w402 = tag "Dev2/ctr0" ("counter")
          w318 = 1000.0 ("frequency")
          w409 = u32 1 ("number of signals")
          w410 = u8 0 items=["0", "1", "Z", "L", "H", "X", "T", "V"] ("value")
          w411 = u8 1 items=["0", "1", "Z", "L", "H", "X", "T", "V"] ("value")
          w412 = u8 0 items=["0", "1", "Z", "L", "H", "X", "T", "V"] ("value")
          w420 = 1 items=["one channel for each line", "one channel for all lines"] ("line grouping")
          w294 = 10123 items=["Finite Samples"=10178, "Continuous Samples"=10123] ("sample mode")
          # "Default valve signal"
          # "Create trigger signal"
          # "Create Valve signal"
          n135 = Equal?(x=0, y=w362) -> (x = y?=w356:bool)
          n136 = flat-sequence {
            tunnel: [w468] -> w339
            tunnel: w357 -> [w468]
            tunnel: w356 -> [w467]
            tunnel: w355 -> [w466]
            tunnel: w354 -> [w465]
            tunnel: [w464] -> w353
            tunnel: [w461] -> w343
            tunnel: w337 -> [w460]
            tunnel: w335 -> [w459]
            frame #0 {
              n137 = case shown="True" w467 {
                tunnel: [w470 w471] -> w464
                tunnel: w466 -> [w470 _]
                tunnel: w465 -> [_ w480]
                tunnel: w460 -> [_ w474]
                tunnel: [w469 w473] -> w461
                tunnel: w459 -> [w469 _]
                frame False {
                }
                frame True {
                  n138 = property on="Valve order list" class="Arr (strict)"() -> ("Value"=w478:i8[])  [unwired: 2 in, 2 out]
                  n139 = flat-sequence {
                    tunnel: w474 -> [w483]
                    tunnel: [w481] -> w472
                    tunnel: [w485] -> w473
                    tunnel: w472 -> [w485]
                    tunnel: [w484] -> w471
                    frame #0 {
                      n140 = call "CheckFile.vi"("Image count filepath"=w483) -> ("Byte Stream File out"=w482:refnum<file>)  [unwired: 10 in]
                      n141 = call "WriteOdorFileheader.vi"("Byte Stream File in"=w482) -> ("Byte Stream File out"=w481:refnum<file>)  [unwired: 10 in]
                    }
                    frame #1 {
                      n142 = Tick Count (ms)() -> (millisecond timer value=w484:u32)
                    }
                  }
                  n143 = local read "Time between trials"() -> (w475:u16)
                  n144 = Array Size(array=w478) -> (size(s)=w477:i32)
                  n145 = Add(x=w475, y=w480) -> (x+y=w476:dbl)
                  n146 = Multiply(x=w476, y=w477) -> (x*y=→"Estimated total time":dbl)
                }
              }
              n147 = local write "Pause elapsed time"(0.0 ("Pause elapsed time")) -> ()
              n148 = local write "In between trials"(FALSE ("In between trials")) -> ()
              n149 = local write "Trial elapsed time"(0.0 ("Trial elapsed time")) -> ()
            }
          }
          n150 = local read "Total trial time"() -> (w354:dbl)
          n151 = Add(x=i8 16, y=w339) -> (x+y=w394:i8)
          n152 = Number To Decimal String(number=w394) -> (decimal integer string=w395:string)  [unwired: 1 in]
          n153 = Add(x=i8 16, y="Selected default valve") -> (x+y=w306:u8)
          n154 = Number To Decimal String(number=w306) -> (decimal integer string=w305:string)  [unwired: 1 in]
          n155 = Concatenate Strings("/Dev2/port0/line" ("string"), w395) -> (w310:string)
          n156 = Concatenate Strings("/Dev2/port0/line" ("string"), w305) -> (w303:string)
          n157 = case shown="True" "Use Default vavle" {
            tunnel: w310 -> [w430 w433]
            tunnel: "/Dev2/port0/line25" ("string") -> [w429 w432]
            tunnel: [w428 w434] -> w308
            tunnel: w303 -> [_ w431]
            frame False {
              n158 = Build Array(w430, w429) -> (w428:string[])
            }
            frame True {
              n159 = Build Array(w433, w431, w432) -> (w434:string[])
            }
          }
          n160 = local read "Valve opening Time"() -> (w368:dbl)
          n161 = local read "Valve delay"() -> (w367:dbl)
          n162 = call <vilib>:"DAQmx Flatten Channel String.vi"("names in"=w308) -> ("names out"=w384:string, "error out"=w352:errorcluster)  [unwired: 13 in]
          n163 = call-poly <vilib>:"DAQmx Create Virtual Channel.vi"("edge"=w350, "counter"=tag "Dev2/ctr1") -> ("task out"=w333:refnum<k21>, "error out"=w330:errorcluster)  [unwired: 12 in]
          n164 = Add(x=w367, y=w368) -> (x+y=w398:dbl)
          n165 = call-poly <vilib>:"DAQmx Create Virtual Channel.vi"("frequency"=w318, "duty cycle"=0.5, "counter"=w402) -> ("task out"=w423:refnum<k21>, "error out"=w297:errorcluster)  [unwired: 11 in]
          n166 = call-poly <vilib>:"DAQmx Create Virtual Channel.vi"("lines"=w384, "line grouping"=w420, "error in"=w352) -> ("task out"=w427:refnum<k21>, "error out"=w426:errorcluster)  [unwired: 11 in]
          n167 = Concatenate Strings("/", w402, "InternalOutput" ("string")) -> (w349:string)
          n168 = Subtract(x=w354, y=w398) -> (x-y=w397:dbl)
          n169 = Multiply(x=w318, y=w368) -> (x*y=w400:dbl)
          n170 = Multiply(x=w318, y=w367) -> (x*y=w401:dbl)
          n171 = Subtract(x=w354, y=w383) -> (x-y=w392:dbl)
          n172 = Multiply(x=w318, y=w383) -> (x*y=w388:dbl)
          n173 = To Unsigned Long Integer(number=w401) -> (unsigned 32bit integer=w315:u32)
          n174 = Multiply(x=w318, y=w397) -> (x*y=w399:dbl)
          n175 = To Unsigned Long Integer(number=w400) -> (unsigned 32bit integer=w316:u32)
          n176 = Multiply(x=w318, y=w392) -> (x*y=w390:dbl)
          n177 = To Unsigned Long Integer(number=w388) -> (unsigned 32bit integer=w389:u32)
          n178 = To Unsigned Long Integer(number=w399) -> (unsigned 32bit integer=w317:u32)
          n179 = property class="DAQmx Channel"(reference=w333, error in=w330, "CI.CountEdges.Term"=tag "/Dev2/PFI1") -> (reference out=w332:refnum<k21>, error out=w331:errorcluster)
          n180 = To Unsigned Long Integer(number=w390) -> (unsigned 32bit integer=w391:u32)
          n181 = property class="DAQmx Channel"(reference=w423, error in=w297, "CO.Pulse.Term"=tag "/Dev2/PFI12") -> (reference out=w298:refnum<k21>, error out=w296:errorcluster)
          n182 = call-poly <vilib>:"Digital Pattern Generator.vi"("value"=w386, "sample rate"=w318, "number of signals"=w385, "number of samples"=w389) -> ("digital waveform"=w371:digitalwaveform)  [unwired: 6 in, 1 out]
          n183 = call-poly <vilib>:"Digital Pattern Generator.vi"("value"=w321, "sample rate"=w318, "number of signals"=w319, "number of samples"=w316) -> ("digital waveform"=w326:digitalwaveform)  [unwired: 6 in, 1 out]
          n184 = call-poly <vilib>:"Digital Pattern Generator.vi"("value"=w320, "sample rate"=w318, "number of signals"=w319, "number of samples"=w315) -> ("digital waveform"=w327:digitalwaveform)  [unwired: 6 in, 1 out]
          n185 = call-poly <vilib>:"Digital Pattern Generator.vi"("value"=w411, "sample rate"=w318, "number of signals"=w409, "number of samples"=w316) -> ("digital waveform"=w376:digitalwaveform)  [unwired: 6 in, 1 out]
          n186 = call-poly <vilib>:"Digital Pattern Generator.vi"("value"=w412, "sample rate"=w318, "number of signals"=w409, "number of samples"=w315) -> ("digital waveform"=w375:digitalwaveform)  [unwired: 6 in, 1 out]
          n187 = Compound Arithmetic op=ADD(w368, w367, 10.0 ("Wert")) -> (w369:dbl)
          n188 = property on="Digitaler output" class="DigitalGraph (strict)"("XScale.Maximum"=w369) -> ()  [unwired: 2 in, 2 out]
          n189 = call-poly <vilib>:"Digital Pattern Generator.vi"("value"=w387, "sample rate"=w318, "number of signals"=w385, "number of samples"=w391) -> ("digital waveform"=w372:digitalwaveform)  [unwired: 6 in, 1 out]
          n190 = property on="Digital Waveform Graph" class="DigitalGraph (strict)"("XScale.Maximum"=w369) -> ()  [unwired: 2 in, 2 out]
          n191 = call-poly <vilib>:"Digital Pattern Generator.vi"("value"=w322, "sample rate"=w318, "number of signals"=w319, "number of samples"=w317) -> ("digital waveform"=w329:digitalwaveform)  [unwired: 6 in, 1 out]
          n192 = call-poly <vilib>:"Append Digital Samples.vi"("digital waveform B"=w326, "digital waveform A"=w327) -> ("digital waveform out"=w328:digitalwaveform)  [unwired: 8 in, 1 out]
          n193 = call-poly <vilib>:"Digital Pattern Generator.vi"("value"=w410, "sample rate"=w318, "number of signals"=w409, "number of samples"=w317) -> ("digital waveform"=w373:digitalwaveform)  [unwired: 6 in, 1 out]
          n194 = call-poly <vilib>:"Append Digital Samples.vi"("digital waveform B"=w376, "digital waveform A"=w375) -> ("digital waveform out"=w374:digitalwaveform)  [unwired: 8 in, 1 out]
          n195 = disable-structure shown="Enabled" {
            disable-tunnel: w332 -> [w449 w451]
            disable-tunnel: w318 -> [w448 _]
            disable-tunnel: w349 -> [w447 _]
            disable-tunnel: w331 -> [w446 w450]
            disable-tunnel: [w445 w451] -> w348
            disable-tunnel: [w444 w450] -> w292
            disable-tunnel: w294 -> [w443 _]
            frame Enabled {
              n196 = call-poly <vilib>:"DAQmx Timing.vi"("task/channels in"=w449, "sample mode"=w443, "rate"=w448, "source"=w447, "error in"=w446) -> ("task out"=w445:refnum<k21>, "error out"=w444:errorcluster)  [unwired: 9 in]
            }
            frame Disabled {
            }
          }
          n197 = Multiply(x=w354, y=w318) -> (x*y=w289:dbl)
          n198 = call-poly <vilib>:"Append Digital Samples.vi"("digital waveform B"=w372, "digital waveform A"=w371) -> ("digital waveform out"=w382:digitalwaveform)  [unwired: 8 in, 1 out]
          n199 = call-poly <vilib>:"DAQmx Timing.vi"("task/channels in"=w427, "sample mode"=w290, "samples per channel"=w289, "rate"=w318, "source"=w349, "error in"=w426) -> ("task out"=w417:refnum<k21>, "error out"=w416:errorcluster)  [unwired: 8 in]
          n200 = call-poly <vilib>:"Append Digital Samples.vi"("digital waveform B"=w329, "digital waveform A"=w328) -> ("digital waveform out"=w323:digitalwaveform)  [unwired: 8 in, 1 out]
          n201 = call-poly <vilib>:"Append Digital Samples.vi"("digital waveform B"=w373, "digital waveform A"=w374) -> ("digital waveform out"=w379:digitalwaveform)  [unwired: 8 in, 1 out]
          n202 = call-poly <vilib>:"DAQmx Timing.vi"("task/channels in"=w298, "sample mode"=w294, "error in"=w296) -> ("task out"=w421:refnum<k21>, "error out"=w422:errorcluster)  [unwired: 11 in]
          n203 = Set Waveform Attribute(5:"Scanimage trigger", 6:"NI_LineNames" ("name"), 7:w382) -> (3:w312:digitalwaveform)  [unwired: 1 in, 2 out]
          n204 = Set Waveform Attribute(5:"Default Valve signal", 6:"NI_LineNames" ("name"), 7:w323) -> (3:w311:digitalwaveform)  [unwired: 1 in, 2 out]
          n205 = Set Waveform Attribute(5:"Valve signal", 6:"NI_LineNames" ("name"), 7:w379) -> (3:w313:digitalwaveform)  [unwired: 1 in, 2 out]
          n206 = case shown="False" "Use Default vavle" {
            tunnel: w313 -> [w437 w442]
            tunnel: w312 -> [w436 w440]
            tunnel: [w435 w441] -> w314
            tunnel: w311 -> [_ w439]
            frame False {
              n207 = call-poly <vilib>:"Append Digital Signals.vi"("digital waveform (low bits)"=w436, "digital waveform (high bits)"=w437) -> ("digital waveform out"=w435:digitalwaveform)  [unwired: 8 in, 1 out]
            }
            frame True {
              n208 = call-poly <vilib>:"Append Digital Signals.vi"("digital waveform (low bits)"=w440, "digital waveform (high bits)"=w439) -> ("digital waveform out"=w438:digitalwaveform)  [unwired: 8 in, 1 out]
              n209 = call-poly <vilib>:"Append Digital Signals.vi"("digital waveform (low bits)"=w438, "digital waveform (high bits)"=w442) -> ("digital waveform out"=w441:digitalwaveform)  [unwired: 8 in, 1 out]
            }
          }
          n210 = call-poly <vilib>:"DAQmx Write.vi"("task/channels in"=w417, "auto start"=FALSE, "data"=w314, "error in"=w416) -> ("task out"=w415:refnum<k21>, "error out"=w414:errorcluster)  [unwired: 9 in, 1 out]
          n211 = call <vilib>:"DAQmx Start Task.vi"("task/channels in"=w348, "error in"=w292) -> ("task out"=w293:refnum<k21>, "error out"=w291:errorcluster)  [unwired: 12 in]
          n212 = call <vilib>:"DAQmx Start Task.vi"("task/channels in"=w415, "error in"=w414) -> ("task out"=w419:refnum<k21>, "error out"=w418:errorcluster)  [unwired: 12 in]
          n213 = flat-sequence {
            tunnel: [w593] -> w425
            tunnel: [w592] -> w424
            tunnel: w422 -> [w591]
            tunnel: w421 -> [w594]
            tunnel: [w603] -> w408
            tunnel: w419 -> [w603]
            tunnel: [w602] -> w407
            tunnel: w418 -> [w602]
            tunnel: [w601] -> w360
            tunnel: w293 -> [w600]
            tunnel: w291 -> [w599]
            tunnel: [w600] -> w347
            tunnel: [w599] -> w346
            tunnel: bool[] [FALSE, FALSE, FALSE] ("data") -> [w598]
            tunnel: [w598] -> w344
            tunnel: [w597] -> w342
            tunnel: w343 -> [w597]
            tunnel: [w596] -> w340
            tunnel: w308 -> [w596]
            tunnel: [w595] -> w338
            tunnel: w339 -> [w595]
            frame #0 {
              n214 = Tick Count (ms)() -> (millisecond timer value=w601:u32)
              n215 = call <vilib>:"DAQmx Start Task.vi"("task/channels in"=w594, "error in"=w591) -> ("task out"=w593:refnum<k21>, "error out"=w592:errorcluster)  [unwired: 12 in]
            }
          }
          n216 = call-poly <vilib>:"Digital to Boolean Array.vi"("digital waveform"=w314) -> ()  [unwired: 9 in, 2 out]
          n217 = disable-structure shown="Aktiviert" {
            disable-tunnel: w425 -> [w533 _]
            disable-tunnel: w424 -> [w532 _]
            disable-tunnel: [w531 _] -> w364
            disable-tunnel: [w530 _] -> w365
            disable-tunnel: w408 -> [w529 _]
            disable-tunnel: w407 -> [w528 _]
            disable-tunnel: [w527 _] -> w406
            disable-tunnel: [w526 _] -> w359
            disable-tunnel: w360 -> [w525 _]
            disable-tunnel: w353 -> [w524 _]
            disable-tunnel: w347 -> [w514 _]
            disable-tunnel: w346 -> [w523 _]
            disable-tunnel: w344 -> [w522 _]
            disable-tunnel: w342 -> [w521 _]
            disable-tunnel: [w520 _] -> w341
            disable-tunnel: w340 -> [w519 _]
            disable-tunnel: w338 -> [w518 _]
            disable-tunnel: [w517 _] -> w336
            disable-tunnel: [w516 _] -> w334
            disable-tunnel: [w515 _] -> w299
            frame Enabled {
              n218 = while {
                shift-right: [w571] -> w530
                shift-left: w533 -> [w573]
                shift-right: [w570] -> w531
                shift-left: w532 -> [w572]
                tunnel: w529 -> [w569]
                tunnel: w528 -> [w554]
                tunnel: [w540] -> w527
                tunnel: [w538] -> w526
                tunnel: w525 -> [w564]
                tunnel: w524 -> [w561]
                tunnel: w514 -> [w553]
                tunnel: w523 -> [w551]
                tunnel: [w552] -> w515
                tunnel: [w550] -> w520
                shift-right: [w546] -> _
                shift-left: w522 -> [w549]
                shift-right: [w544] -> w517
                shift-left: w521 -> [w545]
                tunnel: w519 -> [w543]
                tunnel: w518 -> [w542]
                tunnel: [w541] -> w516
                stop <- w565 stop-if-true
                n219 = call-poly <vilib>:"DAQmx Read.vi"("task/channels in"=w553, "number of samples per channel"=100, "error in"=w551) -> ("task out"=w552:refnum<k21>, "data"=w534:u32[], "error out"=w550:errorcluster)  [unwired: 10 in]
                n220 = Index Array(array=w534) -> (element=w535:u32)  [unwired: 1 in]
                "Framecount" <- w535
                n221 = call-poly <vilib>:"DAQmx Read.vi"("task/channels in"=w569, "error in"=w554) -> ("task out"=w555:refnum<k21>, "data"=w546:bool[], "error out"=w539:errorcluster)  [unwired: 11 in]
                n222 = Not Equal?(x=w546, y=w549) -> (x != y?=w548:bool[])
                n223 = Or Array Elements(Boolean array=w548) -> (logical OR=w547:bool)
                n224 = Tick Count (ms)() -> (millisecond timer value=w562:u32)
                n225 = case shown="True" w547 {
                  tunnel: w546 -> [_ w587]
                  tunnel: w535 -> [_ w585]
                  tunnel: w545 -> [w576 w589]
                  tunnel: [w576 w588] -> w544
                  tunnel: w543 -> [_ w579]
                  tunnel: w542 -> [_ w582]
                  tunnel: [errorcluster {"status"=FALSE, "code"=0, "source"=""} ("error out") w578] -> w541
                  frame False {
                  }
                  frame True {
                    w580 = "\t"
                    n226 = Boolean To (0,1)(Boolean=w587) -> (0, 1=w586:i16[])
                    n227 = Number To Decimal String(number=w586) -> (decimal integer string=w583:string[])  [unwired: 1 in]
                    n228 = Number To Decimal String(number=w585) -> (decimal integer string=w584:string)  [unwired: 1 in]
                    n229 = Number To Decimal String(number=w582) -> (decimal integer string=w581:string)  [unwired: 1 in]
                    n230 = Concatenate Strings(w584, w580, w583, w580, w581, w580, w579, "\r\n") -> (w590:string)
                    n231 = Write to Text File(file (use dialog)=w589, text=w590) -> (refnum out=w588:refnum<file>, error out=w578:errorcluster)  [unwired: 2 in, 1 out]
                  }
                }
                n232 = Wait (ms)(milliseconds to wait=u32 1 ("Zu wartende ms")) -> ()  [unwired: 1 out]
                n233 = call <vilib>:"DAQmx Is Task Done.vi"("task/channels in"=w555, "error in"=w539) -> ("task out"=w540:refnum<k21>, "task done?"=w537:bool, "error out"=w538:errorcluster)  [unwired: 11 in]
                n234 = Subtract(x=w562, y=w564) -> (x-y=w557:u32)
                n235 = local read "Stop Boolesch"() -> (w566:bool)
                n236 = call <vilib>:"DAQmx Is Task Done.vi"("task/channels in"=w573, "error in"=w572) -> ("task out"=w571:refnum<k21>, "error out"=w570:errorcluster)  [unwired: 11 in, 1 out]
                n237 = Subtract(x=w562, y=w561) -> (x-y=w559:u32)
                n238 = Divide(x=w557, y=u32 1000 ("x")) -> (x/y=→"Trial elapsed time":dbl)
                n239 = Unbundle By Name(w538) -> ("status"=w567:bool)
                n240 = Divide(x=w559, y=u32 1000 ("x")) -> (x/y=→"Total elapsed time":dbl)
                n241 = Or(x=w567, y=w566) -> (x .or. y?=w574:bool)
                n242 = Or(x=w537, y=w574) -> (x .or. y?=w565:bool)
              }
            }
            frame Disabled {
            }
          }
          n243 = local write "Digital Waveform Graph"(w314) -> ()
          n244 = local write "Digitaler output"(w314) -> ()
          n245 = disable-structure shown="Enabled" {
            disable-tunnel: w406 -> [w455 w457]
            disable-tunnel: [w454 w457] -> w363
            disable-tunnel: w359 -> [w453 w456]
            disable-tunnel: [w452 w456] -> w358
            frame Enabled {
              n246 = call <vilib>:"DAQmx Wait Until Done.vi"("task/channels in"=w455, "error in"=w453) -> ("task out"=w454:refnum<k21>, "error out"=w452:errorcluster)  [unwired: 12 in]
            }
            frame Disabled {
            }
          }
          n247 = flat-sequence {
            tunnel: w365 -> [w498]
            tunnel: w364 -> [w487]
            tunnel: w363 -> [w497]
            tunnel: w358 -> [w489]
            tunnel: w341 -> [w492]
            tunnel: w299 -> [w495]
            tunnel: w353 -> [w501]
            frame #0 {
              n248 = call <vilib>:"DAQmx Stop Task.vi"("task/channels in"=w495, "error in"=w492) -> ("task out"=w494:refnum<k21>, "error out"=w493:errorcluster)  [unwired: 12 in]
              n249 = call <vilib>:"DAQmx Stop Task.vi"("task/channels in"=w497, "error in"=w489) -> ("task out"=w490:refnum<k21>, "error out"=w488:errorcluster)  [unwired: 12 in]
              n250 = call <vilib>:"DAQmx Stop Task.vi"("task/channels in"=w498, "error in"=w487) -> ("task out"=w491:refnum<k21>, "error out"=w486:errorcluster)  [unwired: 12 in]
              n251 = call <vilib>:"DAQmx Clear Task.vi"("task in"=w494, "error in"=w493) -> ("error out"=w496:errorcluster)  [unwired: 13 in]
              n252 = call <vilib>:"DAQmx Clear Task.vi"("task in"=w491, "error in"=w486) -> ("error out"=w499:errorcluster)  [unwired: 13 in]
              n253 = call <vilib>:"DAQmx Clear Task.vi"("task in"=w490, "error in"=w488) -> ("error out"=w500:errorcluster)  [unwired: 13 in]
              n254 = Merge Errors(w499, w500, w496) -> ()  [unwired: 1 out]
            }
            frame #1 {
              n255 = Tick Count (ms)() -> (millisecond timer value=w502:u32)
              n256 = for {
                N: "Time between trials" -> [_]
                tunnel: w502 -> [w512]
                tunnel: w501 -> [w507]
                stop <- w505 stop-if-true
                w509 = u32 1000 ("Zu wartende ms")
                n257 = Tick Count (ms)() -> (millisecond timer value=w506:u32)
                n258 = Subtract(x=w506, y=w512) -> (x-y=w513:u32)
                n259 = Subtract(x=w506, y=w507) -> (x-y=w510:u32)
                n260 = local read "Stop Boolesch"() -> (w505:bool)
                n261 = Divide(x=w513, y=w509) -> (x/y=→"Pause elapsed time":dbl)
                n262 = Divide(x=w510, y=w509) -> (x/y=w508:dbl)
                n263 = local write "Total elapsed time"(w508) -> ()
                n264 = Wait (ms)(milliseconds to wait=w509) -> ()  [unwired: 1 out]
              }
              "In between trials" <- TRUE ("In between trials")
            }
          }
          n265 = local read "Stop Boolesch"() -> (w366:bool)
          "Current Valve" <- w357
          "Current list index" <- w362
        }
        n266 = local write "Experiment running"(TRUE ("Experiment running")) -> ()
        n267 = Close File(refnum=w281, error in=w280) -> ()  [unwired: 2 out]
        "State" <- w286
      }
      frame "Stop" {
        n268 = local write "State"(w604) -> ()
        n269 = flat-sequence {
          frame #0 {
            # "Stop-all to zero"
            # "all lines also trigger line"
            n270 = call-poly <vilib>:"DAQmx Write.vi"("task/channels in"="/Dev2/port0/line17:25" ("string"), "data"=bool[] [FALSE, FALSE, FALSE, FALSE, FALSE, FALSE, FALSE, FALSE, FALSE]) -> ("task out"=w612:refnum<k21>, "error out"=w607:errorcluster)  [unwired: 11 in, 1 out]
            n271 = call <vilib>:"DAQmx Start Task.vi"("task/channels in"=w612, "error in"=w607) -> ("task out"=w611:refnum<k21>, "error out"=w609:errorcluster)  [unwired: 12 in]
            n272 = call <vilib>:"DAQmx Wait Until Done.vi"("task/channels in"=w611, "error in"=w609) -> ("task out"=w610:refnum<k21>, "error out"=w608:errorcluster)  [unwired: 12 in]
            n273 = call <vilib>:"DAQmx Clear Task.vi"("task in"=w610, "error in"=w608) -> ()  [unwired: 13 in, 1 out]
          }
          frame #1 {
            w615 = T2."Enabled" ("Deaktiviert")
            n274 = property on="Select experiment" class="TabCtl (strict)"() -> ("Pages"=w618:refnum<vi>[])  [unwired: 2 in, 2 out]
            n275 = property on="Valve order list" class="Arr (strict)"("DisabledEnum"=T2."Enabled" ("Deaktiviert")) -> ()  [unwired: 2 in, 2 out]
            n276 = for {
              tunnel: w618 -> [w619] mode=indexing
              n277 = property class="Page"(reference=w619, "PageEnb"=T3."Page Enabled" ("Aktiv-Status der Seite")) -> ()  [unwired: 1 in, 2 out]
            }
            n278 = property on="Start trial series" class="Bool"("DisabledEnum"=w615) -> ()  [unwired: 2 in, 2 out]
            n279 = property on="Start single trial" class="Bool"("DisabledEnum"=w615) -> ()  [unwired: 2 in, 2 out]
            n280 = property on="Image count filepath" class="Path"("DisabledEnum"=w615) -> ()  [unwired: 2 in, 2 out]
            "Experiment running" <- FALSE ("Experiment running")
          }
        }
        n281 = local read "Stop Boolesch"() -> (w606:bool)
      }
    }
  }
  n282 = while {
    tunnel: w4 -> [w622]
    stop <- w621 stop-if-true
    n283 = event shown="[2] \"Stopp\": Value Change" {
      selector: _ -> [_ _ _ _]
      dyn-events: _ -> [_ _ _ _]
      timeout: _ -> [_ _ _ _]
      tunnel: w622 -> [_ w623 w632 w638]
      event Timeout {
        n284 = event-data() -> ()  [unwired: 1 in, 3 out]
      }
      event "Start single trial": Value Change {
        n285 = event-data() -> ()  [unwired: 1 in, 6 out]
        n286 = case shown="True" "Start single trial" {
          tunnel: w623 -> [_ w631]
          frame False {
          }
          frame True {
            n287 = property on="Start single trial" class="Bool"("DisabledEnum"=T2."Disabled and Grayed Out" ("Deaktiviert")) -> ()  [unwired: 2 in, 2 out]
            n288 = Enqueue Element(queue=w631, element=StatesEnum."Start Trial" ("Enum")) -> ()  [unwired: 2 in, 3 out]
            n289 = property on="Select experiment" class="TabCtl (strict)"() -> ("Pages"=w627:refnum<vi>[])  [unwired: 2 in, 2 out]
            n290 = Index Array(array=w627, index=1 ("Index")) -> (element=w628:refnum<vi>)
            n291 = property class="Page"(reference=w628, "PageEnb"=T3."Page Disabled & Grayed" ("Aktiv-Status der Seite")) -> ()  [unwired: 1 in, 2 out]
          }
        }
      }
      event "Stopp": Value Change {
        n292 = event-data() -> ()  [unwired: 1 in, 6 out]
        n293 = case shown="True" "Stopp" {
          tunnel: w632 -> [_ w636]
          frame False {
          }
          frame True {
            n294 = Enqueue Element(queue=w636, element=StatesEnum."Stop" ("Enum")) -> ()  [unwired: 2 in, 3 out]
            "Stop Boolesch" <- TRUE ("Stop Boolesch")
          }
        }
      }
      event "Start trial series": Value Change {
        n295 = event-data() -> ()  [unwired: 1 in, 6 out]
        n296 = case shown="True" "Start trial series" {
          tunnel: w638 -> [_ w645]
          frame False {
          }
          frame True {
            n297 = property on="Start trial series" class="Bool"("DisabledEnum"=T2."Disabled and Grayed Out" ("Deaktiviert")) -> ()  [unwired: 2 in, 2 out]
            n298 = Enqueue Element(queue=w645, element=StatesEnum."Start trial series" ("Enum")) -> ()  [unwired: 2 in, 3 out]
            n299 = property on="Select experiment" class="TabCtl (strict)"() -> ("Pages"=w641:refnum<vi>[])  [unwired: 2 in, 2 out]
            n300 = Index Array(array=w641, index=0 ("Index")) -> (element=w642:refnum<vi>)
            n301 = property class="Page"(reference=w642, "PageEnb"=T3."Page Disabled & Grayed" ("Aktiv-Status der Seite")) -> ()  [unwired: 1 in, 2 out]
          }
        }
      }
    }
    n302 = local read "Stop Boolesch"() -> (w621:bool)
  }
  n303 = Release Queue(queue=w3) -> ()  [unwired: 2 in, 3 out]
